vi "read_eval_print.vi"(10 "Environment in":T1, 11 "input string":string="(progn\n  (define pi 3.14)\n  (define circle-area \n    (lambda (r)\n      (* r r pi)))\n  (define cylinder-volume \n    (lambda (r h) (* (circle-area r) h)))\n  (cylinder-volume 4 2))\n") -> (2 "Environment out":T1, 3 "expression out":string)   [LabVIEW 2021]
uses:
  Expression.ctl
  ExpressionType.ctl
  Environment.ctl
panel:
  in  "ShowType?":bool=TRUE
  out "Expression in":T2
  out "Expression out":T2
  out "expression in":string
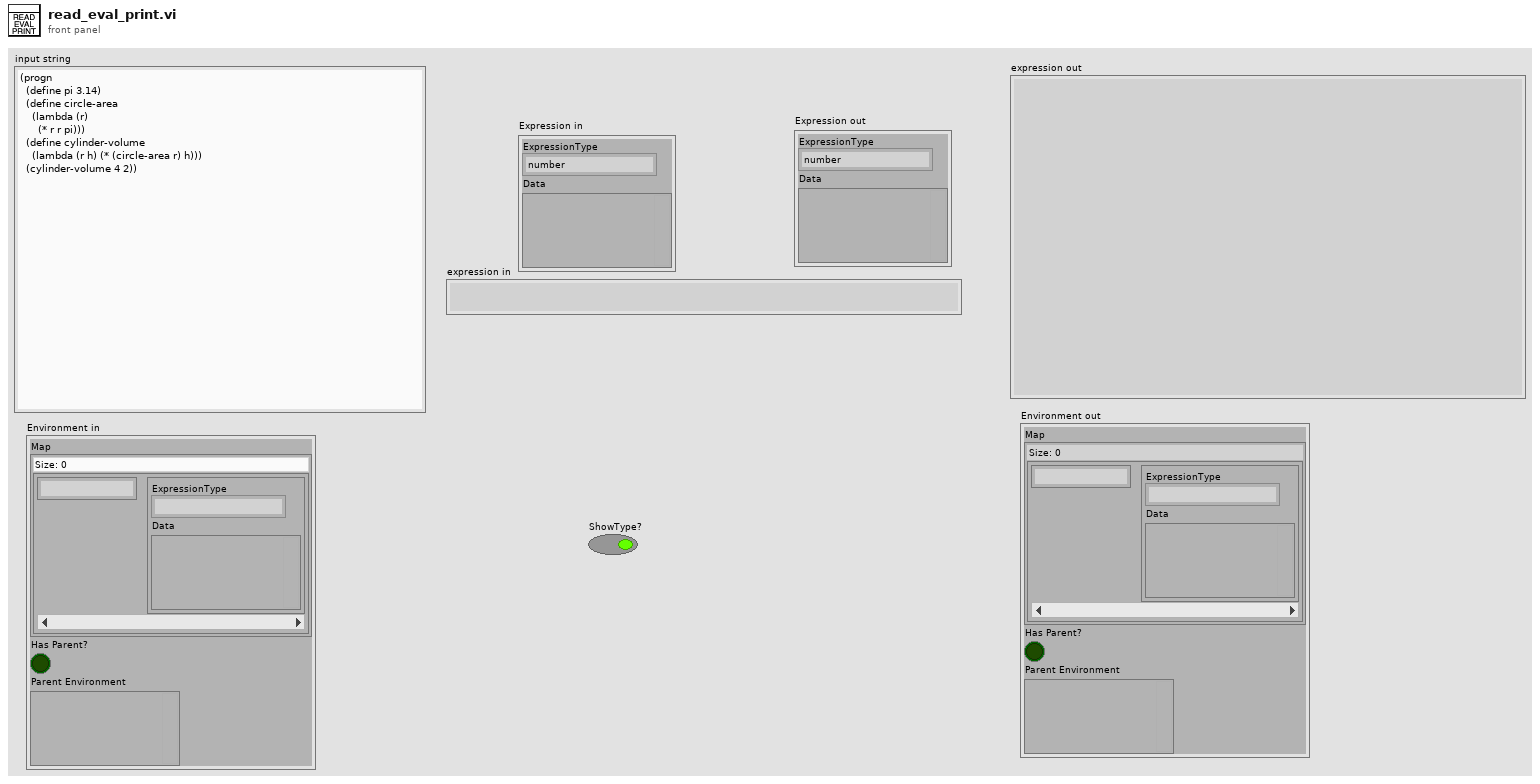
[diagram p1: front panel]
types:
  T1 = typedef "Environment.ctl" = cluster{"Map":map{string, T2}, "Has Parent?":bool, "Parent Environment":variant}
  T2 = typedef "Expression.ctl" = cluster{"ExpressionType":T3, "Data":variant}
  T3 = typedef "ExpressionType.ctl" = enum16{"number", "string", "symbol", "primitive", "list", "closure", "nil", "error"}
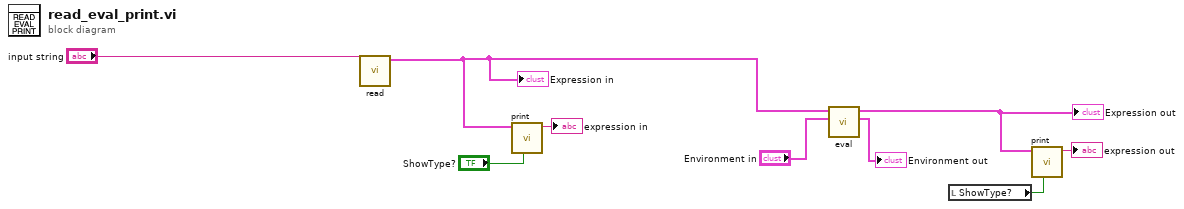
[diagram p0: block diagram]
diagram:
  n1 = call "read.vi"("input string"="input string") -> ("Expression out"=w5:T2)  [unwired: 10 in]
  "Expression in" <- w5
  n2 = call "print.vi"("ShowType?"="ShowType?", "Expression"=w5) -> ("String"=→"expression in":string)  [unwired: 8 in, 1 out]
  n3 = call "eval.vi"("Environment in"="Environment in", "Expression in"=w5) -> ("Environment out"=→"Environment out":T1, "Expression out"=w6:T2)  [unwired: 6 in]
  "Expression out" <- w6
  n4 = local read "ShowType?"() -> (w4:bool)
  n5 = call "print.vi"("ShowType?"=w4, "Expression"=w6) -> ("String"=→"expression out":string)  [unwired: 8 in, 1 out]
